vi "WavelengthScan.vi"(3 "error in (no error)":errorcluster, 4 "End wavelength":u16=1 min=1 step=1, 5 "Start wavelength":u16=1 min=1 step=1, 6 "VISA resource name":refnum<visa-resource-name>) -> (0 "error out":errorcluster, 1 "Command not accepted":bool, 2 "VISA resource name out":refnum<visa-resource-name>)   [LabVIEW 2017, in "Spectral Products CM110.lvlib"]
uses:
  Spectral Products CM110.lvlib
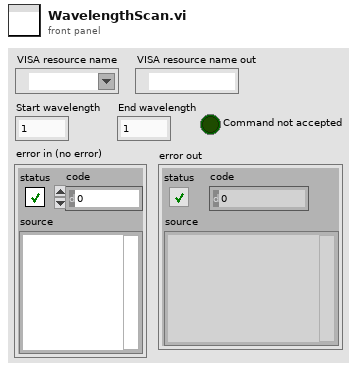
[diagram p1: front panel]
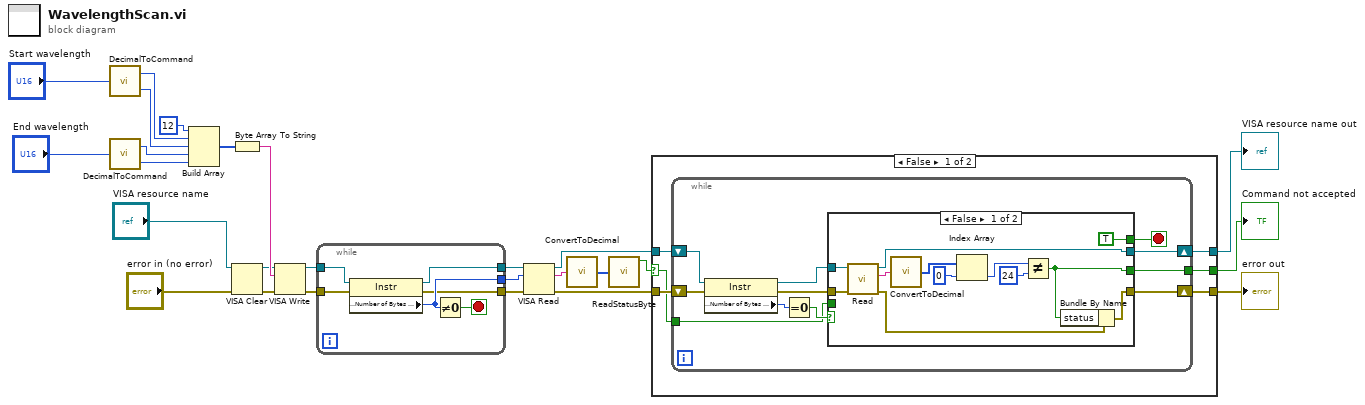
[diagram p0: block diagram]
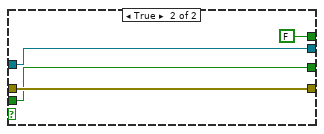
[diagram p2: hidden frame]
diagram:
  n1 = call "DecimalToCommand.vi"("Decimal"="Start wavelength") -> ("HiByte"=w24:u8, "LoByte"=w23:u8)  [unwired: 4 in]
  n2 = call "DecimalToCommand.vi"("Decimal"="End wavelength") -> ("HiByte"=w19:u8, "LoByte"=w18:u8)  [unwired: 4 in]
  n3 = Build Array(u8 12, w24, w23, w19, w18) -> (w22:u8[])
  n4 = Byte Array To String(unsigned byte array=w22) -> (string=w21:string)
  n5 = VISA Clear(VISA resource name="VISA resource name", error in (no error)="error in (no error)") -> (VISA resource name out=w2:refnum<visa-resource-name>, error out=w1:errorcluster)
  n6 = VISA Write(VISA resource name=w2, write buffer=w21, error in (no error)=w1) -> (VISA resource name out=w16:refnum<visa-resource-name>, error out=w15:errorcluster)  [unwired: 1 out]
  n7 = while {
    tunnel: w16 -> [w32]
    tunnel: w15 -> [w31]
    tunnel: [w29] -> w14
    tunnel: [w28] -> w13
    tunnel: [w27] -> w12
    stop <- w30 stop-if-true
    n8 = property class="Instr"(reference=w32, error in=w31) -> (reference out=w28:refnum<visa-resource-name>, error out=w27:errorcluster, "Serial Settings:Number of Bytes at Serial Port"=w29:u32)
    n9 = Not Equal To 0?(x=w29) -> (x != 0?=w30:bool)
  }
  n10 = VISA Read(VISA resource name=w13, byte count=w14, error in (no error)=w12) -> (VISA resource name out=w7:refnum<visa-resource-name>, read buffer=w11:string, error out=w6:errorcluster)  [unwired: 1 out]
  n11 = call "ConvertToDecimal.vi"("read buffer"=w11) -> ("unsigned byte array"=w17:u8[])
  n12 = call "ReadStatusByte.vi"("unsigned byte array"=w17) -> ("Command not accepted"=w5:bool)  [unwired: 4 in, 5 out]
  n13 = case shown="False" w5 {
    selector: w5 -> [w33 w66]
    tunnel: w7 -> [w38 w68]
    tunnel: w6 -> [w37 w67]
    tunnel: [w36 w68] -> w9
    tunnel: [w35 w67] -> w8
    tunnel: [w34 w66] -> w10
    frame False {
      n14 = while {
        shift-right: [w42] -> w36
        shift-left: w38 -> [w49]
        shift-right: [w41] -> w35
        shift-left: w37 -> [w48]
        tunnel: [w40] -> w34
        tunnel: w33 -> [w39]
        stop <- w47 stop-if-true
        n15 = property class="Instr"(reference=w49, error in=w48) -> (reference out=w46:refnum<visa-resource-name>, error out=w45:errorcluster, "Serial Settings:Number of Bytes at Serial Port"=w44:u32)
        n16 = Equal To 0?(x=w44) -> (x = 0?=w43:bool)
        n17 = case shown="False" w43 {
          tunnel: [TRUE FALSE] -> w47
          tunnel: w46 -> [w61 w64]
          tunnel: w45 -> [w60 w63]
          tunnel: [w53 w64] -> w42
          tunnel: [w51 w63] -> w41
          tunnel: [w50 w62] -> w40
          tunnel: w39 -> [_ w62]
          frame False {
            n18 = call "Read.vi"("error in (no error)"=w60, "VISA Refnum in"=w61) -> ("error out"=w52:errorcluster, "read buffer"=w59:string, "VISA Refnum out"=w53:refnum<visa-resource-name>)  [unwired: 6 in, 1 out]
            n19 = call "ConvertToDecimal.vi"("read buffer"=w59) -> ("unsigned byte array"=w58:u8[])
            n20 = Index Array(array=w58, index=0) -> (element=w56:u8)
            n21 = Not Equal?(x=w56, y=u8 24) -> (x != y?=w50:bool)
            n22 = Bundle By Name(cluster=w52, "status"=w50) -> (w51:errorcluster)
          }
          frame True {
          }
        }
      }
    }
    frame True {
    }
  }
  "VISA resource name out" <- w9
  "error out" <- w8
  "Command not accepted" <- w10
